vi "Teleop.vi"(10 "Match Info":T1={"Autonomous Elapsed Seconds"=0.0, "TeleOp Elapsed Seconds"=0.0, "Disabled Elapsed Seconds"=0.0, "Visited Autonomous"=FALSE, "Visited TeleOp"=FALSE, "Visited Disabled"=FALSE, "Autonomous Settings"={"Autonomous Style"=enum."Independent", "VI Refnum"=refnum}}, 11 "Call Context":T2) -> ()   [LabVIEW 2015]
doc: "This VI is called for each TeleOp packet received from the DS where the robot is not disabled. It is often used to read from the joysticks and update I/O or to update setpoints for timed control loops. It should complete and return within 20 milliseconds or it may miss DS packets."
uses:
  <vilib>/Rock Robotics/WPI/DriverStation/WPI_DriverStationDerivedRobotMode.ctl
  <vilib>/Rock Robotics/WPI/DriverStation/WPI_DriverStationMatch Info.ctl
  <vilib>/Rock Robotics/WPI/Solenoid/WPI_SolenoidValue.ctl
  <vilib>/Rock Robotics/WPI/Utilities/WPI_GetSetVariantRefNum.vi
  <vilib>/Rock Robotics/Network Tables/NT Read Boolean.vi
  <vilib>/Rock Robotics/Network Tables/NT Read Number.vi
  <vilib>/Rock Robotics/WPI/Solenoid/WPI_SolenoidSetEnum.vi
  <vilib>/addons/control/pid/NI_PID_pid.lvlib
  <vilib>/addons/control/pid/pid.llb/PID (DBL).vi
panel:
  out "Encodeur gauche max":dbl
  out "Encodeur droit max":dbl
  out "Encodeur gauche min":dbl
  out "Encodeur droit min":dbl
  out "Sample Slider 0":dbl(slide) scale=0.0..5.0
  out "Sample Boolean 1":bool
  out "Sample Boolean 0":bool
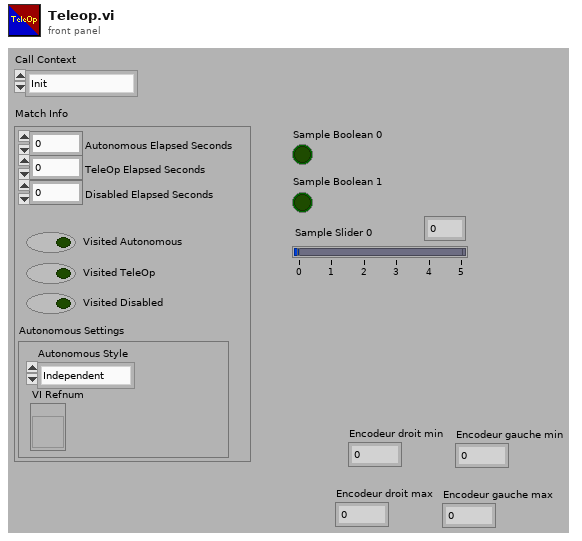
[diagram p1: front panel]
types:
  T1 = typedef "WPI_DriverStationMatch Info.ctl" = cluster{"Autonomous Elapsed Seconds":dbl, "TeleOp Elapsed Seconds":dbl, "Disabled Elapsed Seconds":dbl, "Visited Autonomous":bool, "Visited TeleOp":bool, "Visited Disabled":bool, "Autonomous Settings":cluster{"Autonomous Style":enum16{"Iterative", "Independent"}, "VI Refnum":refnum<vi>}}
  T2 = typedef "WPI_DriverStationDerivedRobotMode.ctl" = enum16{"Init", "Execute", "Stop"}
  T3 = typedef "WPI_JoystickDevRef.ctl" = cluster{"Device":T4}
  T4 = typedef "WPI_JoystickDeviceEnum.ctl" = enum16{"USB 0", "USB 1", "USB 2", "USB 3", "USB 4", "USB 5"}
  T5 = typedef "WPI_EncoderDevRef.ctl" = cluster{"DevStatus":errorcluster, "EncoderIndex":T6, "CounterIndex":T7, "DistancePerCount":dbl, "Decoding Type":T8}
  T6 = typedef "FPGA_EncoderIdx.ctl" = enum8{"Enc 0", "Enc 1", "Enc 2", "Enc 3", "Enc 4", "Enc 5", "Enc 6", "Enc 7", "Invalid"}
  T7 = typedef "FPGA_CounterCtrSystemIndex.ctl" = enum8{"Ctr 0", "Ctr 1", "Ctr 2", "Ctr 3", "Ctr 4", "Ctr 5", "Ctr 6", "Ctr 7", "Invalid"}
  T8 = typedef "WPI_EncoderType.ctl" = enum16{"1x", "2x", "4x"}
  T9 = cluster{"Buttons[0]":bool, "Buttons[1]":bool, "Buttons[2]":bool, "Buttons[3]":bool, "Buttons[4]":bool, "Buttons[5]":bool, "Buttons[6]":bool, "Buttons[7]":bool, "Buttons[8]":bool}
  T10 = cluster{"proportional gain (Kc)":dbl, "integral time (Ti, min)":dbl, "derivative time (Td, min)":dbl}
  T11 = cluster{"Axes[0]":dbl, "Axes[1]":dbl, "Axes[2]":dbl, "Axes[3]":dbl, "Axes[4]":dbl, "Axes[5]":dbl, "Axes[6]":dbl, "Axes[7]":dbl, "Axes[8]":dbl}
  T12 = typedef "WPI_SolenoidDevRef.ctl" = cluster{"DevStatus":errorcluster, "Pneumatics Control Module":u8, "Forward Solenoid Channel":T13, "Reverse Solenoid Channel":T13}
  T13 = typedef "WPI_SolenoidChannel.ctl" = enum8{"Solenoid 0", "Solenoid 1", "Solenoid 2", "Solenoid 3", "Solenoid 4", "Solenoid 5", "Solenoid 6", "Solenoid 7", "Invalid"}
  T14 = typedef "WPI_MotorControlDeviceRef.ctl" = cluster{"DeviceStatus":errorcluster, "Type":T15, "PWM":cluster{"PWM Channel":T16, "DeadBand":T17}, "CAN":cluster{"Device Number":u8, "Control Mode":T18, "Semaphore":T19, "Max Vout":dbl, "TalonSRX Control Mode":T20}, "Invert":bool}
  T15 = typedef "WPI_MotorControlType.ctl" = enum16{"PWM", "CAN", "CANTalonSRX"}
  T16 = typedef "FPGA_DIOPWMChannel.ctl" = enum8{"PWM 0", "PWM 1", "PWM 2", "PWM 3", "PWM 4", "PWM 5", "PWM 6", "PWM 7", "PWM 8", "PWM 9", "PWM MXP 0", "PWM MXP 1", "PWM MXP 2", "PWM MXP 3", "PWM MXP 4", "PWM MXP 5", "PWM MXP 6", "PWM MXP 7", "PWM MXP 8", "PWM MXP 9", "Invalid"}
  T17 = typedef "WPI_PWMDeadband.ctl" = cluster{"Name":string, "maxPositivePwm":i32, "minPositivePwm":i32, "centerPwm":i32, "maxNegativePwm":i32, "minNegativePwm":i32, "angularRange":u16}
  T18 = typedef "WPI_CANJaguar_ControlMode.ctl" = enum8{"Percent VBus", "Current", "Speed", "Position", "Voltage"}
  T19 = typedef "Semaphore RefNum" = refnum<k1>
  T20 = typedef "WPI_CANTalonSRX_APIControlMode.ctl" = enum8{"Percent VBus", "Speed", "Position", "Slave", "Unchanged / Invalid", "Voltage Compensation", "Current", "Motion Profile"}
  T21 = typedef "WPI_SolenoidValue.ctl" = enum16{"Off", "On", "Forward", "Reverse"}
  T22 = typedef "WPI_ServoDeviceRef.ctl" = cluster{"DeviceStatus":errorcluster, "PWM Channel":T16, "DeadBand":T17}
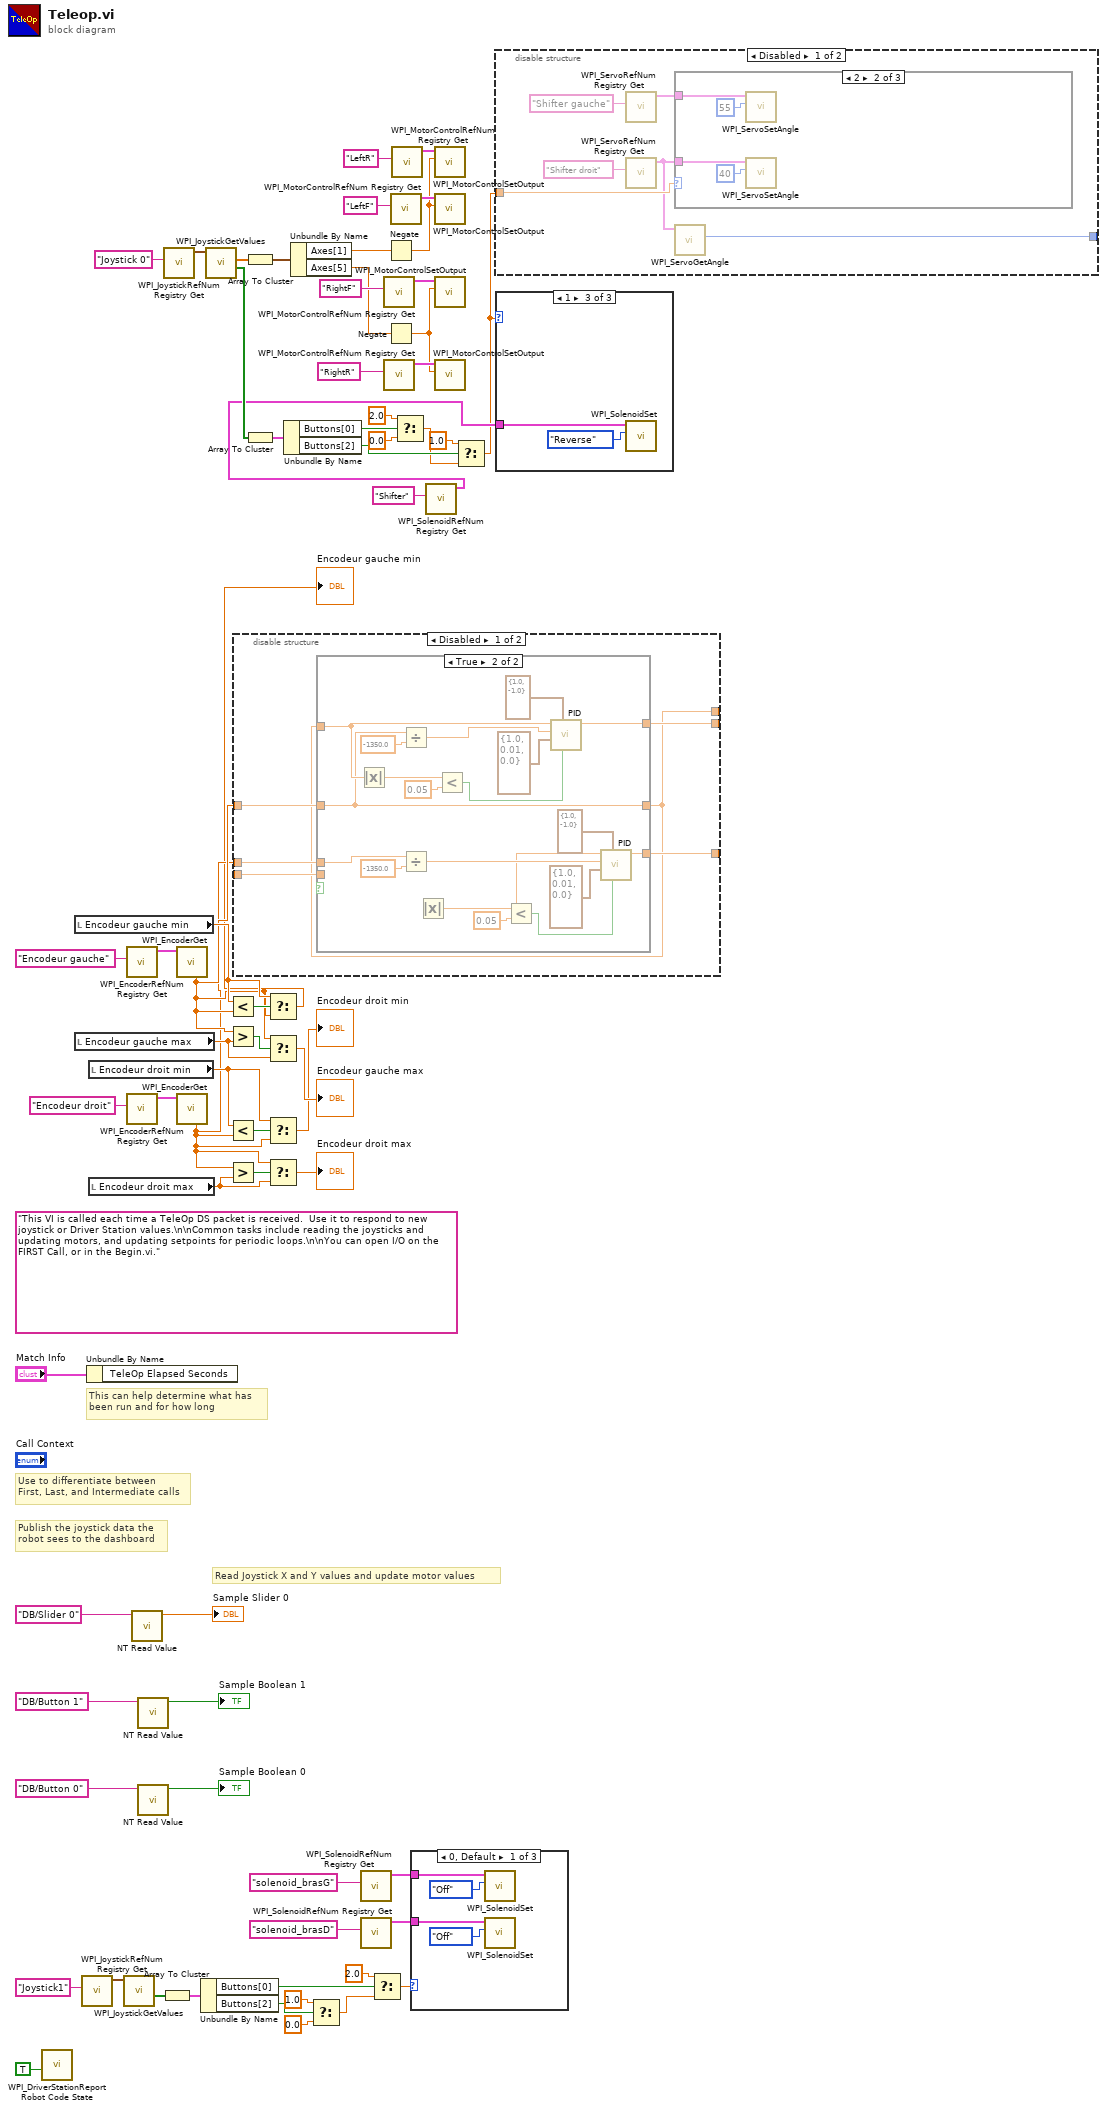
[diagram p0: block diagram]
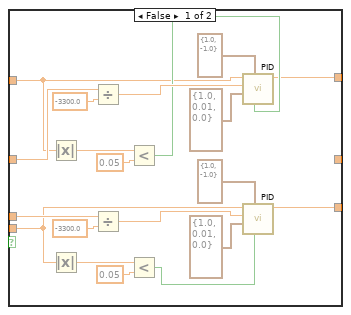
[diagram p2: hidden frame]
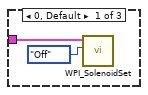
[diagram p4: hidden frame]
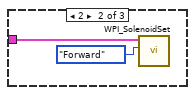
[diagram p5: hidden frame]
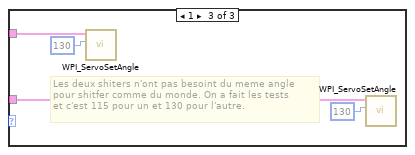
[diagram p7: hidden frame]
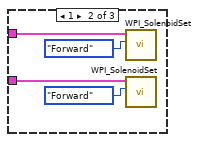
[diagram p9: hidden frame]
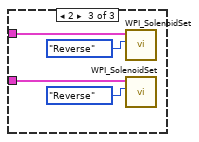
[diagram p10: hidden frame]
diagram:
  (unwired) "This VI is called each time a TeleOp DS packet is received.  Use it to respond to new joystick or Driver Station values.\n\nCommon tasks include reading the joysticks and updating motors, and updating setpoints for periodic loops.\n\nYou can open I/O on the FIRST Call, or in the Begin.vi."
  # "Publish the joystick data the\nrobot sees to the dashboard"
  # "Use to differentiate between\nFirst, Last, and Intermediate calls"
  # "This can help determine what has\nbeen run and for how long"
  # "Read Joystick X and Y values and update motor values"
  n1 = call <vilib>:"WPI_DriverStationReport Robot Code State.vi"("TeleOp"=TRUE ("Autonomous")) -> ()  [unwired: 10 in, 1 out]
  n2 = local read "Encodeur gauche min"() -> (w28:dbl)
  n3 = local read "Encodeur gauche max"() -> (w31:dbl)
  n4 = call <vilib>:"WPI_JoystickRefNum Registry Get.vi"("refnum name"="Joystick1") -> ("JoystickDevRef"=w47:T3)  [unwired: 1 in, 9 out]
  n5 = Unbundle By Name("Match Info") -> ()  [unwired: 1 out]
  n6 = local read "Encodeur droit min"() -> (w24:dbl)
  n7 = local read "Encodeur droit max"() -> (w26:dbl)
  n8 = call <vilib>:"WPI_JoystickGetValues.vi"("JoystickDevRef"=w47) -> ("Buttons"=w48:bool[])  [unwired: 6 in, 4 out]
  n9 = call <vilib>:"WPI_EncoderRefNum Registry Get.vi"("refnum name"="Encodeur gauche") -> ("EncoderDevRef"=w34:T5)  [unwired: 9 in, 1 out]
  n10 = call <vilib>:"WPI_EncoderRefNum Registry Get.vi"("refnum name"="Encodeur droit") -> ("EncoderDevRef"=w35:T5)  [unwired: 9 in, 1 out]
  n11 = call-poly <vilib>:"NT Read Value.vi"("Name"="DB/Slider 0" ("refnum name")) -> ("Numeric"=→"Sample Slider 0":dbl)  [unwired: 9 in, 1 out]
  n12 = call-poly <vilib>:"NT Read Value.vi"("Name"="DB/Button 1" ("refnum name")) -> ("Boolean"=→"Sample Boolean 1":bool)  [unwired: 9 in, 1 out]
  n13 = call-poly <vilib>:"NT Read Value.vi"("Name"="DB/Button 0" ("refnum name")) -> ("Boolean"=→"Sample Boolean 0":bool)  [unwired: 9 in, 1 out]
  n14 = Array To Cluster(array=w48) -> (cluster=w49:T9)
  n15 = call <vilib>:"WPI_JoystickRefNum Registry Get.vi"("refnum name"="Joystick 0") -> ("JoystickDevRef"=w66:T3)  [unwired: 1 in, 9 out]
  n16 = call <vilib>:"WPI_EncoderGet.vi"("EncoderDevRef"=w34) -> ("Rate"=w13:dbl)  [unwired: 5 in, 5 out]
  n17 = call <vilib>:"WPI_EncoderGet.vi"("EncoderDevRef"=w35) -> ("Rate"=w12:dbl)  [unwired: 5 in, 5 out]
  n18 = Unbundle By Name(w49) -> ("Buttons[0]"=w43:bool, "Buttons[2]"=w42:bool)
  n19 = call <vilib>:"WPI_JoystickGetValues.vi"("JoystickDevRef"=w66) -> ("Buttons"=w58:bool[], "Axes"=w60:dbl[])  [unwired: 6 in, 3 out]
  n20 = Less?(x=w28, y=w13) -> (x < y?=w29:bool)
  n21 = Greater?(x=w13, y=w31) -> (0:w32:bool)
  n22 = Less?(x=w24, y=w12) -> (x < y?=w25:bool)
  n23 = Greater?(x=w12, y=w26) -> (0:w27:bool)
  n24 = disable-structure shown="Disabled" {
    disable-tunnel: w13 -> [w70 _]
    disable-tunnel: [w74 _] -> _
    disable-tunnel: [w69 _] -> _
    disable-tunnel: _ -> [w73 _]
    disable-tunnel: w12 -> [w72 _]
    disable-tunnel: [w71 _] -> _
    frame Disabled {
      n25 = case shown="True" {
        selector: _ -> [_ _]
        tunnel: w69 -> [w76 w106]
        tunnel: [w80 w107] -> w74
        tunnel: w73 -> [w75 _]
        tunnel: w72 -> [w77 w98]
        tunnel: [w79 w97] -> w71
        tunnel: w70 -> [w78 w95]
        tunnel: [_ w95] -> w69
        frame False {
          n26 = Absolute Value(x=w76) -> (abs(x)=w93:dbl)
          n27 = Absolute Value(x=w75) -> (abs(x)=w86:dbl)
          n28 = Divide(x=w78, y=-3300.0) -> (x/y=w91:dbl)
          n29 = Divide(x=w77, y=-3300.0) -> (x/y=w84:dbl)
          n30 = Less?(x=w93, y=0.05) -> (x < y?=w81:bool)
          n31 = Less?(x=w86, y=0.05) -> (x < y?=w88:bool)
          n32 = call-poly <vilib>:"PID.vi"("reinitialize? (F)"=w81, "output range"=cluster{"output high":dbl, "output low":dbl} {"output high"=1.0, "output low"=-1.0}, "PID gains"=T10 {"proportional gain (Kc)"=1.0, "integral time (Ti, min)"=0.01, "derivative time (Td, min)"=0.0}, "process variable"=w91, "setpoint"=w76) -> ("output"=w80:dbl)  [unwired: 5 in, 1 out]
          n33 = call-poly <vilib>:"PID.vi"("reinitialize? (F)"=w88, "output range"=cluster{"output high":dbl, "output low":dbl} {"output high"=1.0, "output low"=-1.0}, "PID gains"=T10 {"proportional gain (Kc)"=1.0, "integral time (Ti, min)"=0.01, "derivative time (Td, min)"=0.0}, "process variable"=w84, "setpoint"=w75) -> ("output"=w79:dbl)  [unwired: 5 in, 1 out]
        }
        frame True {
          n34 = Absolute Value(x=w106) -> (abs(x)=w112:dbl)
          n35 = Divide(x=w95, y=-1350.0) -> (x/y=w110:dbl)
          n36 = Divide(x=w98, y=-1350.0) -> (x/y=w101:dbl)
          n37 = Less?(x=w112, y=0.05) -> (x < y?=w114:bool)
          n38 = call-poly <vilib>:"PID.vi"("reinitialize? (F)"=w114, "output range"=cluster{"output high":dbl, "output low":dbl} {"output high"=1.0, "output low"=-1.0}, "PID gains"=T10 {"proportional gain (Kc)"=1.0, "integral time (Ti, min)"=0.01, "derivative time (Td, min)"=0.0}, "process variable"=w110, "setpoint"=w106) -> ("output"=w107:dbl)  [unwired: 5 in, 1 out]
          n39 = Absolute Value(x=w96) -> (abs(x)=w103:dbl)
          n40 = Less?(x=w103, y=0.05) -> (x < y?=w105:bool)
          n41 = call-poly <vilib>:"PID.vi"("reinitialize? (F)"=w105, "output range"=cluster{"output high":dbl, "output low":dbl} {"output high"=1.0, "output low"=-1.0}, "PID gains"=T10 {"proportional gain (Kc)"=1.0, "integral time (Ti, min)"=0.01, "derivative time (Td, min)"=0.0}, "process variable"=w101) -> ("output"=w97:dbl, "setpoint"=w96:dbl)  [unwired: 5 in, 1 out]
        }
      }
    }
    frame Enabled {
    }
  }
  n42 = Array To Cluster(array=w60) -> (cluster=w59:T11)
  n43 = Array To Cluster(array=w58) -> (cluster=w57:T9)
  n44 = Select(t=w28, s=w29, f=w13) -> (s? t:f=→"Encodeur gauche min":dbl)
  n45 = Select(t=w13, s=w32, f=w31) -> (s? t:f=→"Encodeur gauche max":dbl)
  n46 = Select(t=w24, s=w25, f=w12) -> (s? t:f=→"Encodeur droit min":dbl)
  n47 = Select(t=w12, s=w27, f=w26) -> (s? t:f=→"Encodeur droit max":dbl)
  n48 = Unbundle By Name(w57) -> ("Buttons[0]"=w56:bool, "Buttons[2]"=w53:bool)
  n49 = Unbundle By Name(w59) -> ("Axes[1]"=w4:dbl, "Axes[5]"=w2:dbl)
  n50 = Select(t=1.0, s=w42, f=0.0) -> (s? t:f=w44:dbl)
  n51 = call <vilib>:"WPI_SolenoidRefNum Registry Get.vi"("refnum name"="solenoid_brasG") -> ("SolenoidDevRef"=w37:T12)  [unwired: 9 in, 1 out]
  n52 = call <vilib>:"WPI_SolenoidRefNum Registry Get.vi"("refnum name"="solenoid_brasD") -> ("SolenoidDevRef"=w5:T12)  [unwired: 9 in, 1 out]
  n53 = Select(t=2.0, s=w43, f=w44) -> (s? t:f=w38:dbl)
  n54 = call <vilib>:"WPI_MotorControlRefNum Registry Get.vi"("refnum name"="RightF") -> ("MotorControlDevRef"=w19:T14)  [unwired: 9 in, 1 out]
  n55 = call <vilib>:"WPI_MotorControlRefNum Registry Get.vi"("refnum name"="RightR") -> ("MotorControlDevRef"=w18:T14)  [unwired: 9 in, 1 out]
  n56 = Negate(x=w4) -> (-x=w3:dbl)
  n57 = Negate(x=w2) -> (-x=w1:dbl)
  n58 = call <vilib>:"WPI_MotorControlRefNum Registry Get.vi"("refnum name"="LeftF") -> ("MotorControlDevRef"=w21:T14)  [unwired: 9 in, 1 out]
  n59 = call <vilib>:"WPI_MotorControlRefNum Registry Get.vi"("refnum name"="LeftR") -> ("MotorControlDevRef"=w20:T14)  [unwired: 9 in, 1 out]
  n60 = Select(t=2.0, s=w56, f=0.0) -> (s? t:f=w52:dbl)
  n61 = case shown="0, Default" w38 {
    tunnel: w37 -> [w117 w122 w125]
    tunnel: w5 -> [w115 w119 w123]
    frame 0, Default {
      n62 = call-poly <vilib>:"WPI_SolenoidSet.vi"("Value"=WPI_SolenoidValue."Off", "SolenoidDevRef"=w117) -> ()  [unwired: 8 in, 2 out]
      n63 = call-poly <vilib>:"WPI_SolenoidSet.vi"("Value"=WPI_SolenoidValue."Off", "SolenoidDevRef"=w115) -> ()  [unwired: 8 in, 2 out]
    }
    frame 1 {
      n64 = call-poly <vilib>:"WPI_SolenoidSet.vi"("Value"=WPI_SolenoidValue."Forward", "SolenoidDevRef"=w122) -> ()  [unwired: 8 in, 2 out]
      n65 = call-poly <vilib>:"WPI_SolenoidSet.vi"("Value"=WPI_SolenoidValue."Forward", "SolenoidDevRef"=w119) -> ()  [unwired: 8 in, 2 out]
    }
    frame 2 {
      n66 = call-poly <vilib>:"WPI_SolenoidSet.vi"("Value"=WPI_SolenoidValue."Reverse", "SolenoidDevRef"=w125) -> ()  [unwired: 8 in, 2 out]
      n67 = call-poly <vilib>:"WPI_SolenoidSet.vi"("Value"=WPI_SolenoidValue."Reverse", "SolenoidDevRef"=w123) -> ()  [unwired: 8 in, 2 out]
    }
  }
  n68 = call <vilib>:"WPI_SolenoidRefNum Registry Get.vi"("refnum name"="Shifter") -> ("SolenoidDevRef"=w10:T12)  [unwired: 9 in, 1 out]
  n69 = call <vilib>:"WPI_MotorControlSetOutput.vi"("Output"=w3, "MotorControlDevRef"=w20) -> ()  [unwired: 7 in, 3 out]
  n70 = call <vilib>:"WPI_MotorControlSetOutput.vi"("Output"=w3, "MotorControlDevRef"=w21) -> ()  [unwired: 7 in, 3 out]
  n71 = call <vilib>:"WPI_MotorControlSetOutput.vi"("Output"=w1, "MotorControlDevRef"=w19) -> ()  [unwired: 7 in, 3 out]
  n72 = call <vilib>:"WPI_MotorControlSetOutput.vi"("Output"=w1, "MotorControlDevRef"=w18) -> ()  [unwired: 7 in, 3 out]
  n73 = Select(t=1.0, s=w53, f=w52) -> (s? t:f=w9:dbl)
  n74 = disable-structure shown="Disabled" {
    disable-tunnel: w9 -> [w129 _]
    disable-tunnel: [w127 _] -> _
    frame Disabled {
      n75 = call <vilib>:"WPI_ServoRefNum Registry Get.vi"("refnum name"="Shifter gauche") -> ("ServoDeviceRef"=w130:T22)  [unwired: 9 in, 1 out]
      n76 = call <vilib>:"WPI_ServoRefNum Registry Get.vi"("refnum name"="Shifter droit") -> ("ServoDeviceRef"=w128:T22)  [unwired: 9 in, 1 out]
      n77 = case shown="2" w129 {
        tunnel: w130 -> [_ w136 w140]
        tunnel: w128 -> [_ w135 w139]
        frame 0, Default {
        }
        frame 2 {
          n78 = call <vilib>:"WPI_ServoSetAngle.vi"("Angle"=55, "ServoDeviceRef"=w136) -> ()  [unwired: 8 in, 2 out]
          n79 = call <vilib>:"WPI_ServoSetAngle.vi"("Angle"=40, "ServoDeviceRef"=w135) -> ()  [unwired: 8 in, 2 out]
        }
        frame 1 {
          # "Les deux shiters n'ont pas besoint du meme angle \npour shitfer comme du monde. On a fait les tests \net c'est 115 pour un et 130 pour l'autre."
          n80 = call <vilib>:"WPI_ServoSetAngle.vi"("Angle"=130, "ServoDeviceRef"=w140) -> ()  [unwired: 8 in, 2 out]
          n81 = call <vilib>:"WPI_ServoSetAngle.vi"("Angle"=130, "ServoDeviceRef"=w139) -> ()  [unwired: 8 in, 2 out]
        }
      }
      n82 = call <vilib>:"WPI_ServoGetAngle.vi"("ServoDeviceRef"=w128) -> ("Angle"=w127:u16)  [unwired: 7 in, 2 out]
    }
    frame Enabled {
    }
  }
  n83 = case shown="1" w9 {
    tunnel: w10 -> [w142 w144 w145]
    frame 0, Default {
      n84 = call-poly <vilib>:"WPI_SolenoidSet.vi"("Value"=WPI_SolenoidValue."Off", "SolenoidDevRef"=w142) -> ()  [unwired: 8 in, 2 out]
    }
    frame 2 {
      n85 = call-poly <vilib>:"WPI_SolenoidSet.vi"("Value"=WPI_SolenoidValue."Forward", "SolenoidDevRef"=w144) -> ()  [unwired: 8 in, 2 out]
    }
    frame 1 {
      n86 = call-poly <vilib>:"WPI_SolenoidSet.vi"("Value"=WPI_SolenoidValue."Reverse", "SolenoidDevRef"=w145) -> ()  [unwired: 8 in, 2 out]
    }
  }
